vi "testpair server2.vi"() -> ()   [LabVIEW 2016]
uses:
  dllwrapper/action complete event.ctl
  tls classes/connection creator/server acceptor/server acceptor.lvclass
  C:/Users/IEUser/Desktop/libasynclvtls/tls classes/connection creator/connection creator.lvclass
  tls classes/engine context/engine context.lvclass
  tls classes/connection/connection.lvclass
  tls classes/connection creator/connection creator.lvclass
  dllwrapper/async tls dl.lvlib
panel:
  out "Numeric":i32
  out "length":i32
  out "error out 3":errorcluster
  out "error out 2":errorcluster
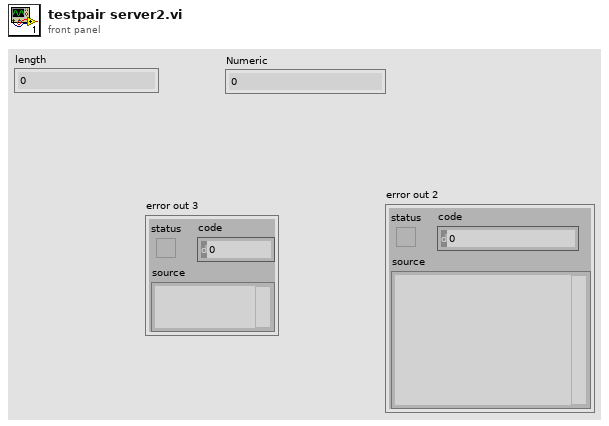
[diagram p1: front panel]
types:
  T1 = typedef "async tls dl.lvlib/action complete event.ctl" = cluster{"request ID":u32, "error code":i32, "error string":string}
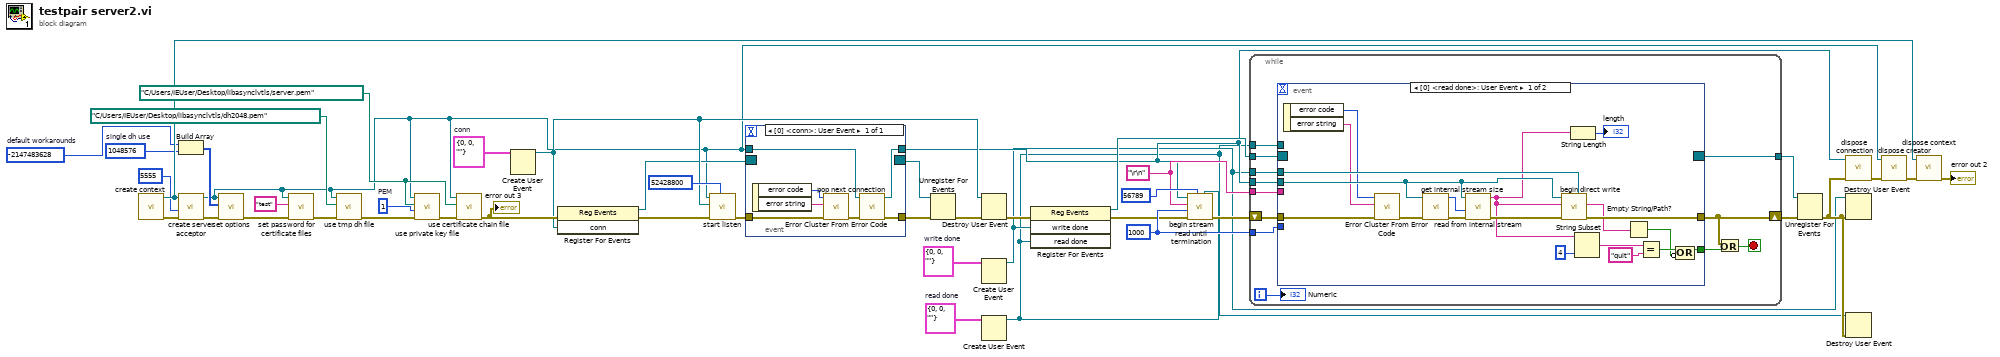
[diagram p0: block diagram]
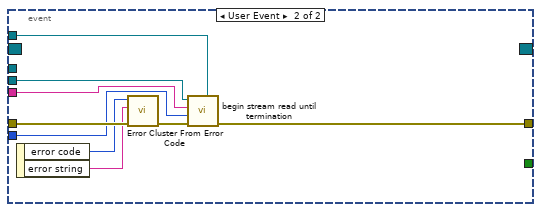
[diagram p2: hidden frame]
diagram:
  w10 = T1 {"request ID"=0, "error code"=0, "error string"=""}  # read done
  w9 = T1 {"request ID"=0, "error code"=0, "error string"=""}  # write done
  w20 = T1 {"request ID"=0, "error code"=0, "error string"=""}  # conn
  w25 = 1  # PEM
  w28 = "\r\n" ("termination")
  w32 = path "C:/Users/IEUser/Desktop/libasynclvtls/server.pem" ("cert chain file")
  w35 = -2147483628  # default workarounds
  w36 = 1048576  # single dh use
  w27 = 1000 ("bytes to read")
  n1 = call "create context.vi"() -> ("error out"=w39:errorcluster, "engine context out"=w38:refnum<class "engine context.lvclass">)  [unwired: 10 in]
  n2 = Build Array(w35, w36) -> (w29:i32[])
  n3 = call "create server acceptor.vi"("error in"=w39, "port"=u16 5555, "engine context in"=w38) -> ("error out"=w37:errorcluster, "server acceptor out"=w4:refnum<class "server acceptor.lvclass">)  [unwired: 7 in]
  n4 = call "set options.vi"("error in"=w37, "options"=w29, "connection creator in"=w4) -> ("error out"=w34:errorcluster)  [unwired: 8 in]
  n5 = call "set password for certificate files.vi"("error in"=w34, "password"="test" ("file"), "connection creator in"=w4) -> ("error out"=w24:errorcluster)  [unwired: 8 in]
  n6 = call "use tmp dh file.vi"("error in"=w24, "tmp dh file"=path "C:/Users/IEUser/Desktop/libasynclvtls/dh2048.pem", "connection creator in"=w4) -> ("error out"=w23:errorcluster)  [unwired: 8 in]
  n7 = call "use private key file.vi"("error in"=w23, "format"=w25, "private key file"=w32, "connection creator in"=w4) -> ("error out"=w22:errorcluster)  [unwired: 7 in]
  n8 = call "use certificate chain file.vi"("error in"=w22, "cert chain file"=w32, "connection creator in"=w4) -> ("error out"=w31:errorcluster)  [unwired: 8 in]
  "error out 3" <- w31
  n9 = Create User Event(user event datatype=w20) -> (user event=w15:refnum<user-event>)  [unwired: 1 in, 1 out]
  n10 = register-events(error in=w31, w15) -> (reference out=w11:refnum<event-registration>, error out=w19:errorcluster)  [unwired: 1 in]
  n11 = call "start listen.vi"("stream buffer size"=u64 52428800, "error in"=w19, "completion event"=w15, "server acceptor in"=w4) -> ("error out"=w13:errorcluster)  [unwired: 7 in]
  n12 = event shown="[0] <conn>: User Event" {
    selector: w11 -> [_]
    dyn-events: [_] -> w12
    timeout: _ -> [_]
    tunnel: [w50] -> w14
    tunnel: w13 -> [w51]
    tunnel: w4 -> [w46]
    tunnel: [w45] -> w3
    event User Event {
      n13 = event-data() -> ("error code"=w48:i32, "error string"=w47:string)  [unwired: 1 in]
      n14 = call <vilib>:"Error Cluster From Error Code.vi"("error in (no error)"=w51, "error message (\"\")"=w47, "error code (0)"=w48) -> ("error out"=w49:errorcluster)  [unwired: 6 in]
      n15 = call "pop next connection.vi"("error in"=w49, "connection creator in"=w46) -> ("error out"=w50:errorcluster, "connection out"=w45:refnum<class "connection.lvclass">)  [unwired: 8 in]
    }
  }
  n16 = Unregister For Events(event registration refnum=w12, error in=w14) -> (error out=w18:errorcluster)
  n17 = Destroy User Event(user event=w15, error in=w18) -> (error out=w17:errorcluster)
  n18 = Create User Event(user event datatype=w9) -> (user event=w2:refnum<user-event>)  [unwired: 1 in, 1 out]
  n19 = Create User Event(user event datatype=w10) -> (user event=w1:refnum<user-event>)  [unwired: 1 in, 1 out]
  n20 = register-events(error in=w17, w2, w1) -> (reference out=w8:refnum<event-registration>, error out=w16:errorcluster)  [unwired: 1 in]
  n21 = call "begin stream read until termination.vi"("event"=w1, "id"=u32 56789, "error in"=w16, "max bytes to read"=w27, "termination"=w28, "connection in"=w3) -> ("error out"=w43:errorcluster)  [unwired: 5 in]
  n22 = while {
    tunnel: w8 -> [w63]
    shift-right: [w58] -> w7
    shift-left: w43 -> [w62]
    tunnel: w3 -> [w61]
    tunnel: w27 -> [w60]
    tunnel: w28 -> [w56]
    tunnel: [w55] -> w5
    tunnel: w2 -> [w54]
    tunnel: w1 -> [w53]
    i -> [w52]
    stop <- w59 stop-if-true
    n23 = event shown="[0] <read done>: User Event" {
      selector: w63 -> [_ _]
      dyn-events: [_ _] -> w55
      timeout: _ -> [_ _]
      tunnel: w62 -> [w75 w91]
      tunnel: w61 -> [w76 w89]
      tunnel: [w80 w90] -> w58
      tunnel: w60 -> [_ w88]
      tunnel: [w68 _] -> w57
      tunnel: w56 -> [_ w87]
      tunnel: w54 -> [w72 _]
      tunnel: w53 -> [_ w86]
      event User Event {
        n24 = event-data() -> ("error code"=w70:i32, "error string"=w69:string)  [unwired: 1 in]
        n25 = call <vilib>:"Error Cluster From Error Code.vi"("error in (no error)"=w75, "error message (\"\")"=w69, "error code (0)"=w70) -> ("error out"=w71:errorcluster)  [unwired: 6 in]
        n26 = call "get internal stream size.vi"("error in"=w71, "connection in"=w76) -> ("error out"=w78:errorcluster, "size"=w79:u64)  [unwired: 8 in]
        n27 = call "read from internal stream.vi"("error in"=w78, "max length"=w79, "connection in"=w76) -> ("error out"=w77:errorcluster, "buffer"=w65:string)  [unwired: 7 in]
        n28 = call "begin direct write.vi"("event"=w72, "error in"=w77, "data"=w65, "connection in"=w76) -> ("error out"=w80:errorcluster, "remaining data"=w67:string)  [unwired: 6 in]
        n29 = String Length(string=w65) -> (length=→"length":i32)
        n30 = String Subset(string=w65, length (rest)=4 ("length (rest)")) -> (substring=w73:string)  [unwired: 1 in]
        n31 = Empty String/Path?(string/path=w67) -> (empty?=w66:bool)
        n32 = Equal?(x=w73, y="quit") -> (x = y?=w81:bool)
        n33 = Compound Arithmetic op=OR(w81, invert w66) -> (w68:bool)
      }
      event User Event {
        n34 = event-data() -> ("error code"=w83:i32, "error string"=w84:string)  [unwired: 1 in]
        n35 = call <vilib>:"Error Cluster From Error Code.vi"("error in (no error)"=w91, "error message (\"\")"=w84, "error code (0)"=w83) -> ("error out"=w85:errorcluster)  [unwired: 6 in]
        n36 = call "begin stream read until termination.vi"("event"=w86, "error in"=w85, "max bytes to read"=w88, "termination"=w87, "connection in"=w89) -> ("error out"=w90:errorcluster)  [unwired: 6 in]
      }
    }
    n37 = Or(x=w58, y=w57) -> (x .or. y?=w59:bool)
    "Numeric" <- w52
  }
  n38 = Unregister For Events(event registration refnum=w5, error in=w7) -> (error out=w6:errorcluster)
  n39 = call "dispose connection.vi"("error in"=w6, "connection in"=w3) -> ("error out"=w42:errorcluster)  [unwired: 9 in]
  n40 = Destroy User Event(user event=w2, error in=w6) -> ()  [unwired: 1 out]
  n41 = Destroy User Event(user event=w1, error in=w6) -> ()  [unwired: 1 out]
  n42 = call "dispose creator.vi"("error in"=w42, "connection creator in"=w4) -> ("error out"=w41:errorcluster)  [unwired: 9 in]
  n43 = call "dispose context.vi"("error in"=w41, "engine context out"=w38) -> ("error out"=→"error out 2":errorcluster)  [unwired: 9 in]
